vi "ShortestPathSelector.vi"(7 "All Lines":T1, 11 "Path taken in":T5[][](array[typedef])) -> (1 "Total Distance":dbl, 3 "Shortest Path":T4[](array[typedef]), 4 "All Distances":dbl[](array[numeric]))   [LabVIEW 2014]
uses:
  Controls/PathControl.ctl
  Controls/ShortestPath.ctl
  Libraries/Map Data Folder/All-Lines.ctl
  Libraries/Map Data Folder/LineCluster.ctl
  Libraries/Map Data Folder/LineConnection.ctl
  Libraries/Map Data Folder/Map Data.lvlib
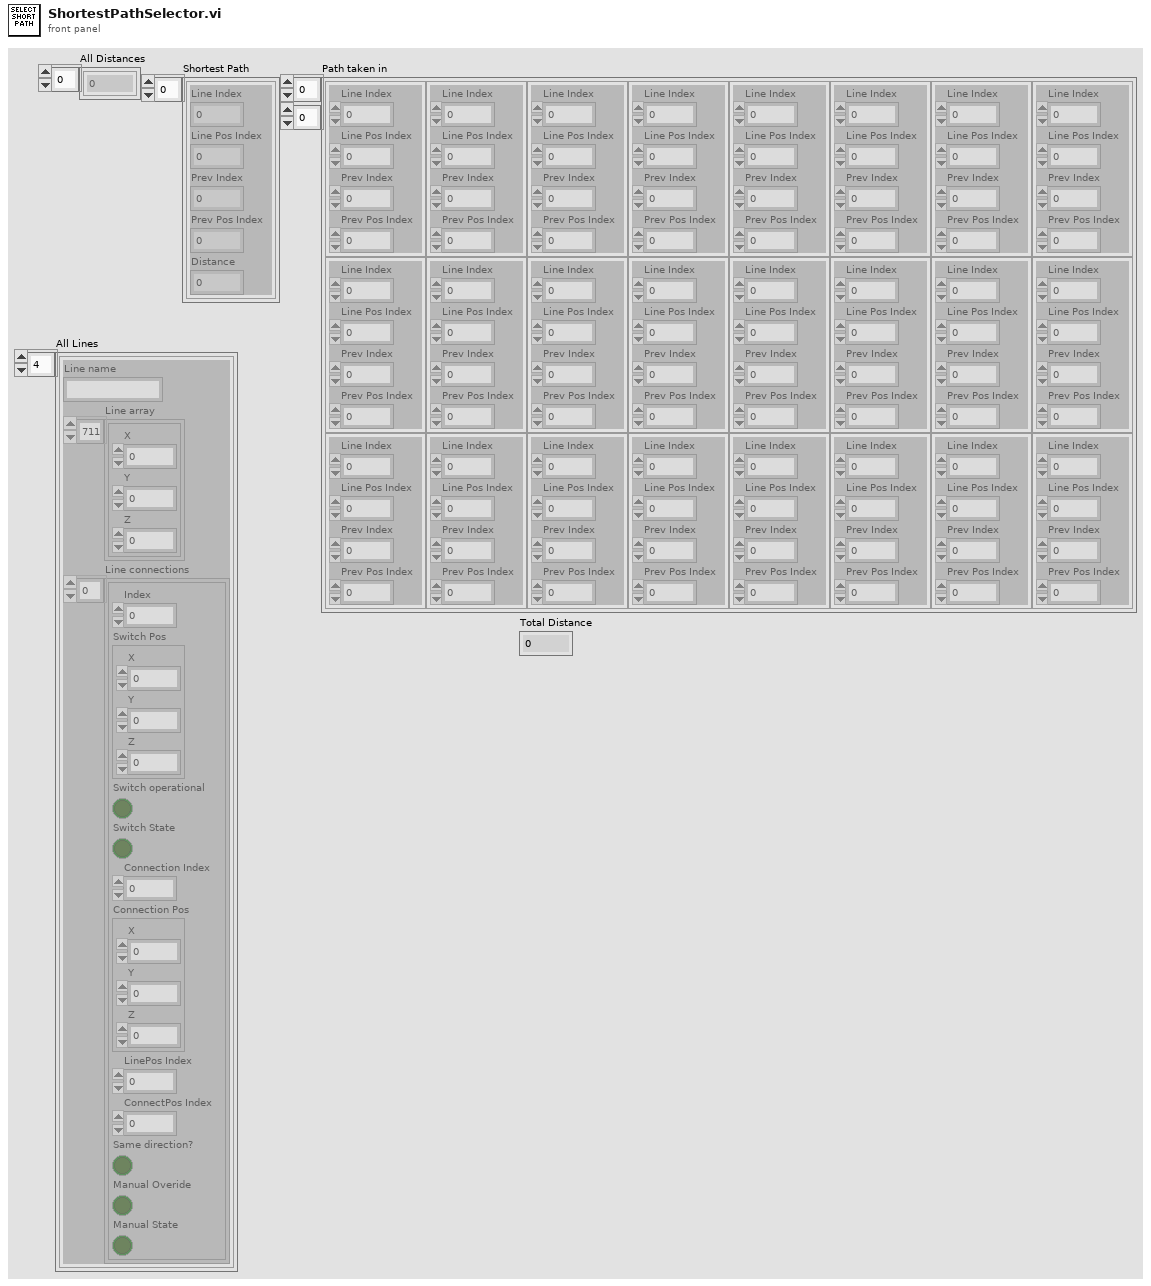
[diagram p1: front panel]
types:
  T1 = typedef "Map Data.lvlib/All-Lines.ctl" = T2[]
  T2 = typedef "Map Data.lvlib/LineCluster.ctl" = cluster{"Line name":string, "Line array":cluster{"X":dbl, "Y":dbl, "Z":dbl}[], "Line connections":T3[]}
  T3 = typedef "Map Data.lvlib/LineConnection.ctl" = cluster{"Index":i32, "Switch Pos":cluster{"X":dbl, "Y":dbl, "Z":dbl}, "Switch operational":bool, "Switch State":bool, "Connection Index":i32, "Connection Pos":cluster{"X":dbl, "Y":dbl, "Z":dbl}, "LinePos Index":i32, "ConnectPos Index":i32, "Same direction?":bool, "Manual Overide":bool, "Manual State":bool}
  T4 = typedef "ShortestPath.ctl" = cluster{"Line Index":i32, "Line Pos Index ":i32, "Prev Index ":i32, "Prev Pos Index":i32, "Distance":dbl}
  T5 = typedef "PathControl.ctl" = cluster{"Line Index":i32, "Line Pos Index ":i32, "Prev Index ":i32, "Prev Pos Index":i32}
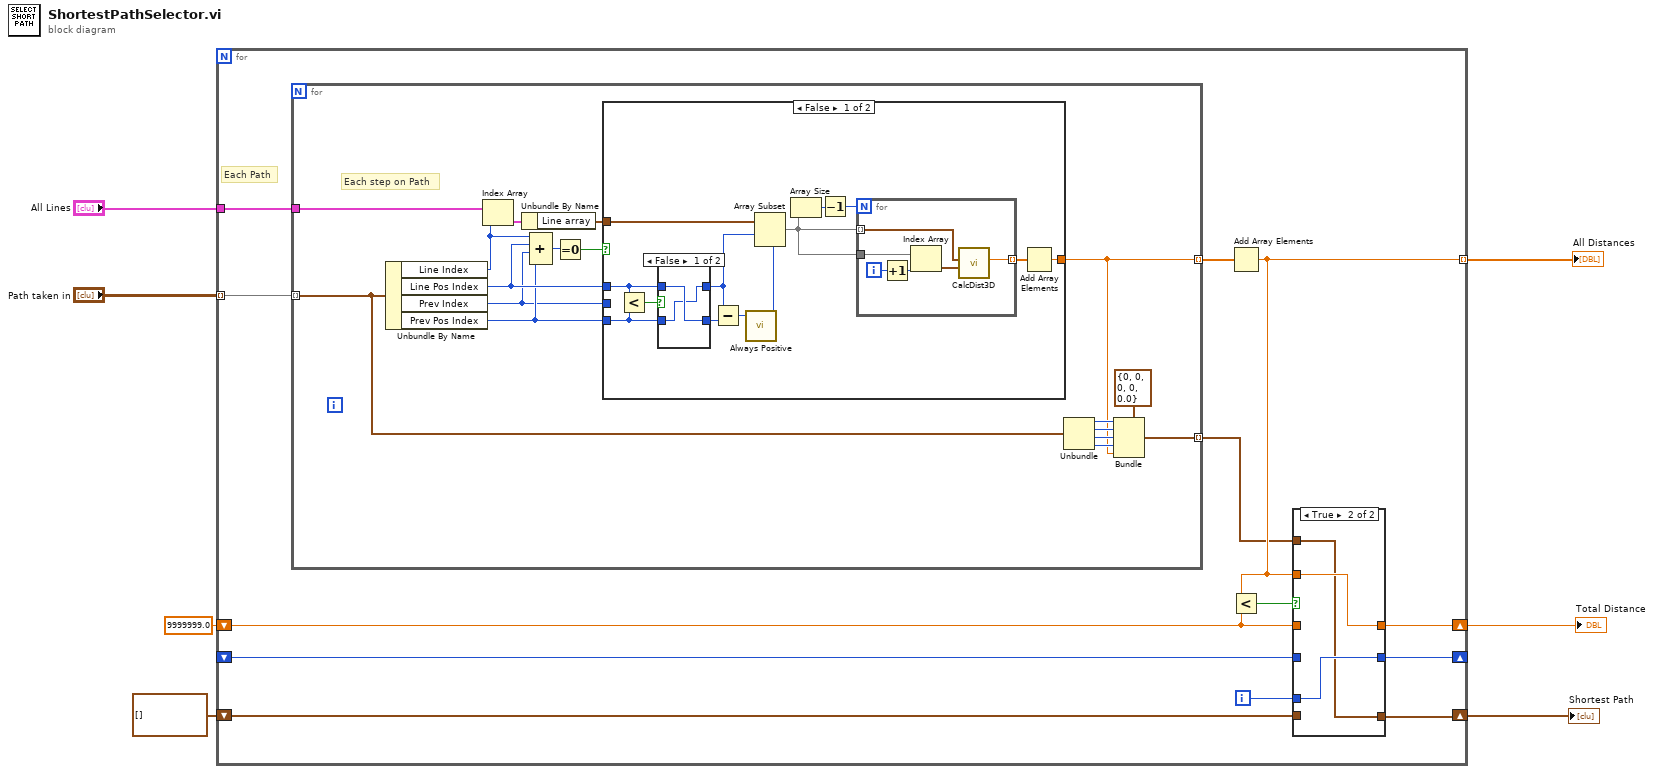
[diagram p0: block diagram]
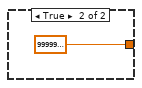
[diagram p4: hidden frame]
diagram:
  n1 = for {
    tunnel: "Path taken in" -> [w14] mode=indexing
    shift-right: [w20] -> w6
    shift-left: 9999999.0 ("Output") -> [w19]
    shift-right: [w17] -> _
    shift-left: _ -> [w15]
    tunnel: "All Lines" -> [w13]
    tunnel: [w11] -> w3 mode=indexing
    shift-right: [w9] -> w1
    shift-left: T4[] [] -> [w8]
    i -> [w16]
    # "Each Path"
    n2 = for {
      tunnel: w14 -> [w29] mode=indexing
      tunnel: [w28] -> w12 mode=indexing
      tunnel: w13 -> [w38]
      tunnel: [w27] -> w10 mode=indexing
      # "Each step on Path"
      n3 = Unbundle By Name(w29) -> ("Line Index"=w37:i32, "Line Pos Index"=w41:i32, "Prev Index"=w39:i32, "Prev Pos Index"=w40:i32)
      n4 = Index Array(array=w38, index=w37) -> (element=w36:T2)
      n5 = Unbundle By Name(w36) -> ("Line array"=w35:cluster{"X":dbl, "Y":dbl, "Z":dbl}[])
      n6 = Compound Arithmetic op=ADD(w37, w41, w39, w40) -> (w43:i32)
      n7 = Equal To 0?(x=w43) -> (x = 0?=w42:bool)
      n8 = case shown="False" w42 {
        tunnel: w40 -> [w49 _]
        tunnel: [w45 999999999.0 ("Distance")] -> w28
        tunnel: w41 -> [w47 _]
        tunnel: w39 -> [_ _]
        tunnel: w35 -> [w56 _]
        frame False {
          n9 = Less?(x=w47, y=w49) -> (x < y?=w51:bool)
          n10 = case shown="False" w51 {
            tunnel: [w58 w60] -> w50
            tunnel: w49 -> [w57 w60]
            tunnel: [w57 w59] -> w48
            tunnel: w47 -> [w58 w59]
            frame False {
            }
            frame True {
            }
          }
          n11 = Subtract(x=w48, y=w50) -> (x-y=w55:i32)
          n12 = call "Always Positive.vi"("Input"=w55) -> ("Output"=w44:i32)  [unwired: 8 in]
          n13 = Array Subset(array=w56, index=w48, length=w44) -> (w54:cluster{"X":dbl, "Y":dbl, "Z":dbl}[])
          n14 = Array Size(array=w54) -> (size(s)=w53:i32)
          n15 = Decrement(x=w53) -> (x-1=w52:i32)
          n16 = for {
            N: w52 -> [_]
            tunnel: w54 -> [w63] mode=indexing
            tunnel: w54 -> [w66]
            tunnel: [w61] -> w46 mode=indexing
            i -> [w65]
            n17 = Increment(x=w65) -> (x+1=w64:i32)
            n18 = Index Array(array=w66, index=w64) -> (element=w62:cluster{"X":dbl, "Y":dbl, "Z":dbl})
            n19 = call "CalcDist3D.vi"("element 2"=w62, "element 1"=w63) -> ("Distance"=w61:dbl)  [unwired: 9 in]
          }
          n20 = Add Array Elements(numeric array=w46) -> (sum=w45:dbl)
        }
        frame True {
        }
      }
      n21 = Unbundle(w29) -> ("Line Index"=w33:i32, "Line Pos Index"=w32:i32, "Prev Index"=w31:i32, "Prev Pos Index"=w30:i32)
      n22 = Bundle(cluster=T4 {"Line Index"=0, "Line Pos Index "=0, "Prev Index "=0, "Prev Pos Index"=0, "Distance"=0.0} ("Posits"), "Line Index"=w33, "Line Pos Index"=w32, "Prev Index"=w31, "Prev Pos Index"=w30, "Distance"=w28) -> (w27:T4)
    }
    n23 = Add Array Elements(numeric array=w12) -> (sum=w11:dbl)
    n24 = Less?(x=w11, y=w19) -> (x < y?=w18:bool)
    n25 = case shown="True" w18 {
      tunnel: w19 -> [w23 _]
      tunnel: [w23 w26] -> w20
      tunnel: w11 -> [_ w26]
      tunnel: [w22 w25] -> w17
      tunnel: w15 -> [w22 _]
      tunnel: w16 -> [_ w25]
      tunnel: w10 -> [_ w24]
      tunnel: [w21 w24] -> w9
      tunnel: w8 -> [w21 _]
      frame False {
      }
      frame True {
      }
    }
  }
  "Shortest Path" <- w1
  "Total Distance" <- w6
  "All Distances" <- w3
